vi "Get All Queues From Registry.vi"(11 "error in":errorcluster) -> (4 "all queues":T2[](array[typedef]), 6 "all properties":T1[](array[typedef]), 10 "number of queues":i32, 15 "error out":errorcluster)   [LabVIEW 2015, in "Car Wash.lvlib" / "AMC.lvlib"]
doc: "Returns all message queue references found in the queue registry."
uses:
  AMC.lvlib
  Queue Registry Method.ctl
  Tools/Keyed Array/KeyedArray.ctl
  Tools/Keyed Array/Tools_KeyedArray.lvlib
  Message.ctl
  Message Queue.ctl
  Queue Registry Properties.ctl
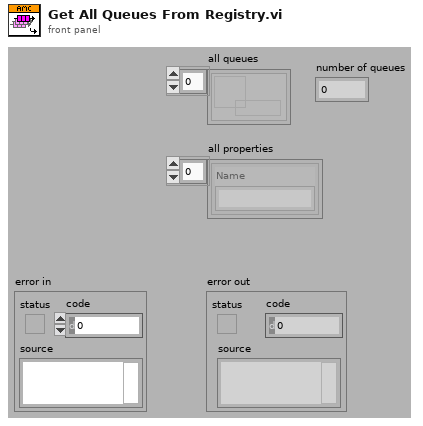
[diagram p1: front panel]
types:
  T1 = typedef "Car Wash.lvlib/AMC.lvlib/Queue Registry Properties.ctl" = cluster{"Name":string}
  T2 = typedef "Car Wash.lvlib/AMC.lvlib/Message Queue.ctl" = refnum<queue>
  T3 = typedef "Car Wash.lvlib/AMC.lvlib/Queue Registry Method.ctl" = enum16{"Initialize", "Add Queue", "Set Properties", "Get Queue by Index", "Get Queue by Name", "Remove Queue", "Remove All Queues"}
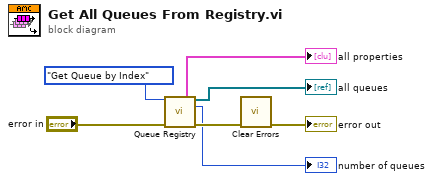
[diagram p0: block diagram]
diagram:
  n1 = call "Queue Registry.vi"("method"=Queue_Registry_Method."Get Queue by Index" ("Method"), "error in"="error in") -> ("all properties"=→"all properties":T1[], "all queues"=→"all queues":T2[], "number of queues"=→"number of queues":i32, "error out"=w5:errorcluster)  [unwired: 8 in, 2 out]
  n2 = call <vilib>:"Clear Errors.vi"("error in (no error)"=w5) -> ("error out"=→"error out":errorcluster)  [unwired: 1 in, 5 out]
